vi "Update UI Interlock.vi"(8 "error in (no error)":errorcluster, 11 "Thermal Chamber Controller In":refnum<class "Thermal Chamber Controller.lvclass">) -> (0 "error out":errorcluster, 3 "Thermal Chamber Controller Out":refnum<class "Thermal Chamber Controller.lvclass">)   [LabVIEW 2020, in "Thermal Chamber Controller.lvclass"]
uses:
  Thermal Chamber Controller.lvclass
  C:/Program Files (x86)/National Instruments/LabVIEW 2020/vi.lib/Asteme/Triarc Framework/Process/Process.lvclass
  <vilib>/Asteme/Triarc Framework/Process/Process.lvclass/Process.ctl
  Thermal Chamber Controller.lvclass/Thermal Chamber Controller.ctl
  <vilib>/Utility/error.llb/Clear Errors.vi
  <vilib>/Asteme/Triarc Framework/Process/Process.lvclass
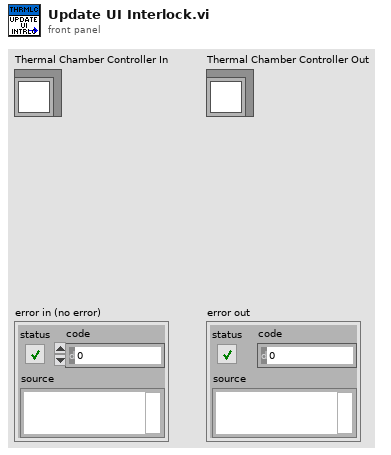
[diagram p1: front panel]
types:
  T1 = enum8{"Enabled", "Disabled", "Disabled and Grayed Out"}
  T2 = typedef "Thermal Chamber Controller.lvclass/Heater State.ctl" = enum16{"Heater Disabled", "Heater Enabled"}
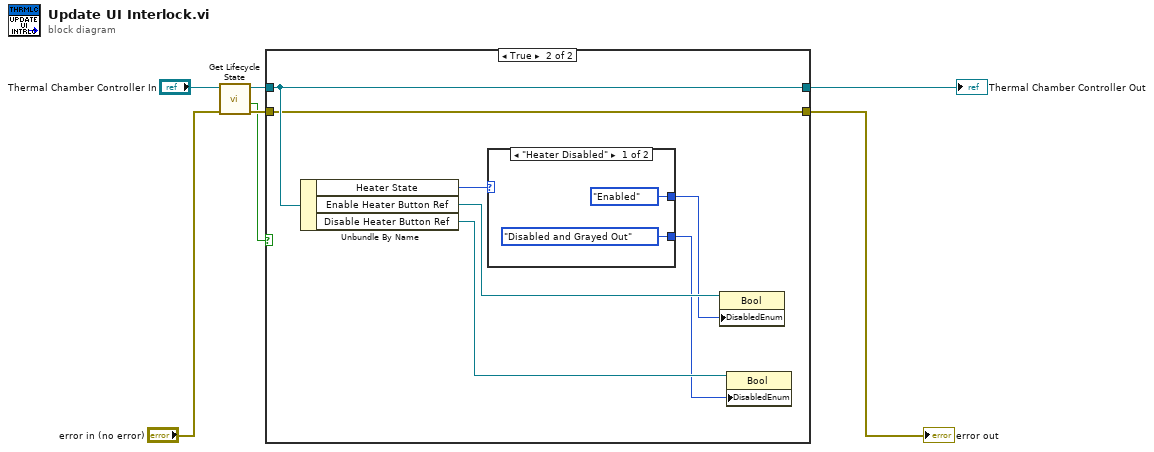
[diagram p0: block diagram]
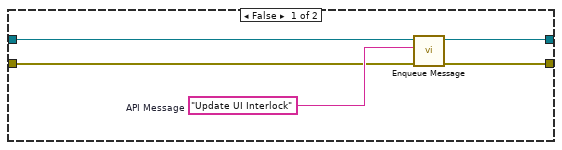
[diagram p2: hidden frame]
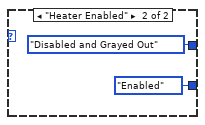
[diagram p3: hidden frame]
diagram:
  n1 = call <vilib>:"Get Lifecycle State.vi"("error in (no error)"="error in (no error)", "Process In"="Thermal Chamber Controller In") -> ("error out"=w4:errorcluster, "In Process Loop?"=w1:bool, "Process Out"=w2:refnum<class "Thermal Chamber Controller.lvclass">)  [unwired: 6 in, 1 out]
  n2 = case shown="True" w1 {
    tunnel: [w12 w19] -> w7
    tunnel: [w11 w18] -> w6
    tunnel: w4 -> [w9 w18]
    tunnel: w2 -> [w8 w19]
    frame False {
      w10 = "Update UI Interlock"  # API Message
      n3 = call <vilib>:"Enqueue Message.vi"("error in (no error)"=w9, "Message"=w10, "Process In"=w8) -> ("error out"=w11:errorcluster, "Process Out"=w12:refnum<class "Thermal Chamber Controller.lvclass">)  [unwired: 7 in]
    }
    frame True {
      n4 = Unbundle By Name(w19) -> ("Heater State"=w16:T2, "Enable Heater Button Ref"=w17:refnum<vi>, "Disable Heater Button Ref"=w15:refnum<vi>)
      n5 = case shown="\"Heater Disabled\"" w16 {
        tunnel: [T1."Enabled" ("Disabled") T1."Disabled and Grayed Out" ("Disabled")] -> w14
        tunnel: [T1."Disabled and Grayed Out" ("Disabled") T1."Enabled" ("Disabled")] -> w13
        frame "Heater Disabled" {
        }
        frame "Heater Enabled" {
        }
      }
      n6 = property class="Bool"(reference=w17, "DisabledEnum"=w14) -> ()  [unwired: 1 in, 2 out]
      n7 = property class="Bool"(reference=w15, "DisabledEnum"=w13) -> ()  [unwired: 1 in, 2 out]
    }
  }
  "error out" <- w6
  "Thermal Chamber Controller Out" <- w7
